vi "Inst_K2002.vi"(8 "error in":errorcluster, 10 "All Message Queues in":T1, 11 "AjustesPrevios in":refnum<class "AjustesPrevios.lvclass">) -> (0 "error out":errorcluster)   [LabVIEW 2019, in "AjustesPrevios.lvclass"]
uses:
  AjustesPrevios.lvclass
  QMH/Message Queue/All Message Queues.ctl
  QMH/Message Queue/Message Cluster.ctl
  AjustesPrevios.lvclass/AjustesPrevios.ctl
  <vilib>/Utility/error.llb/Error Cluster From Error Code.vi
  QMH/Message Queue/Enqueue Message (Single).vi
  <vilib>/ErrorRing/Error Ring.xnode
  QMH/Message Queue/Message Queue.lvlib
  Instrumento/Keithley2002/Keithley2002.lvclass
panel:
  out "All States":string[](array[string])
  out "Actual State":string
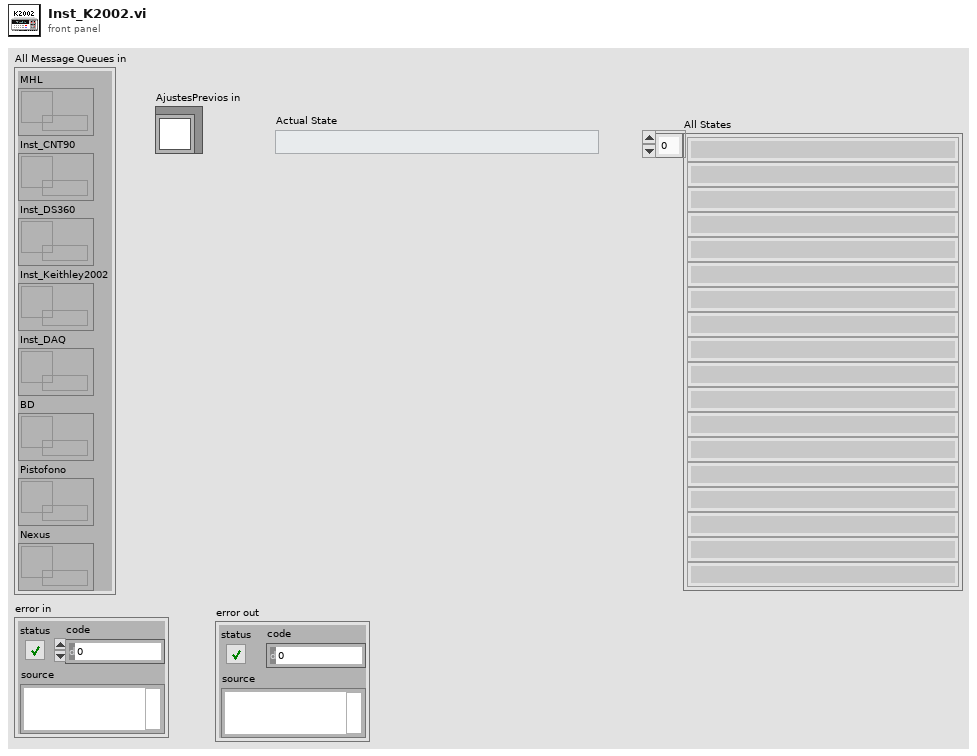
[diagram p1: front panel]
types:
  T1 = typedef "Message Queue.lvlib/All Message Queues.ctl" = cluster{"MHL":refnum<queue>, "Inst_CNT90":refnum<queue>, "Inst_DS360":refnum<queue>, "Inst_Keithley2002":refnum<queue>, "Inst_DAQ":refnum<queue>, "BD":refnum<queue>, "Pistofono":refnum<queue>, "Nexus":refnum<queue>}
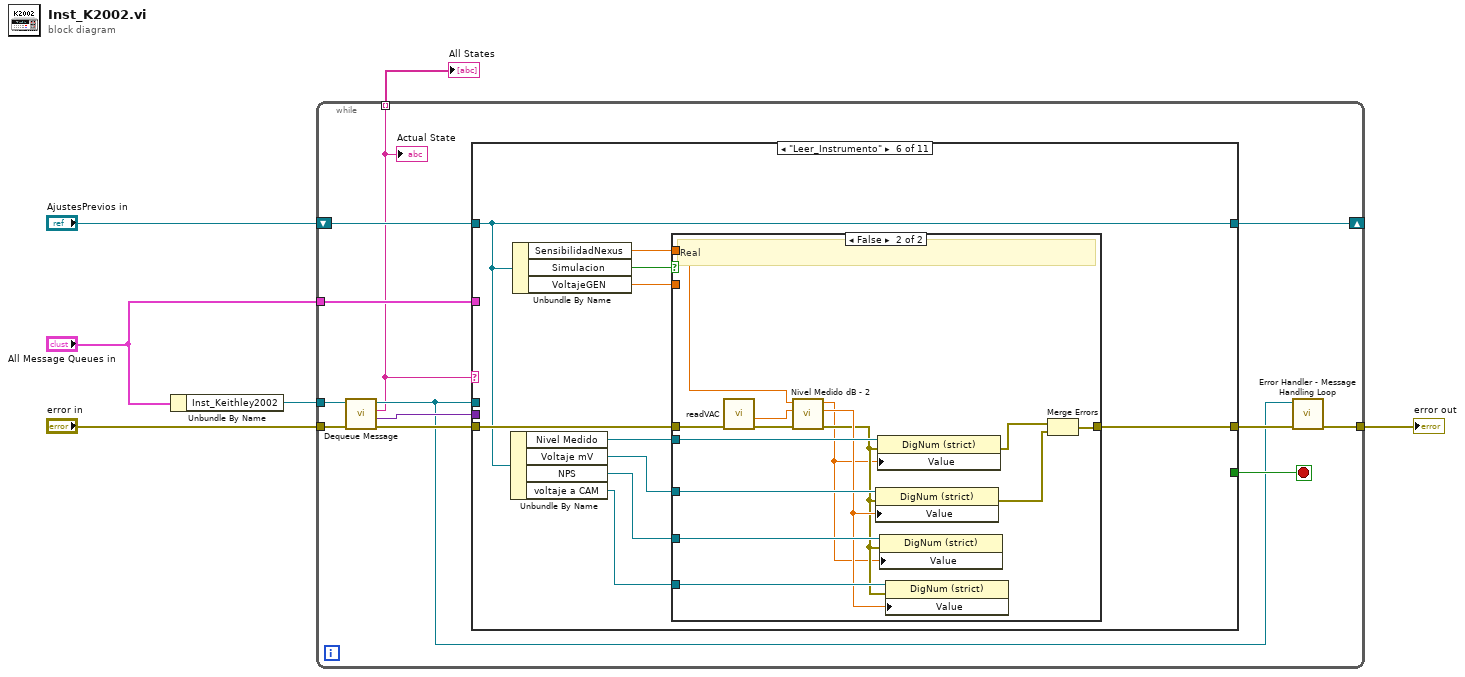
[diagram p0: block diagram]
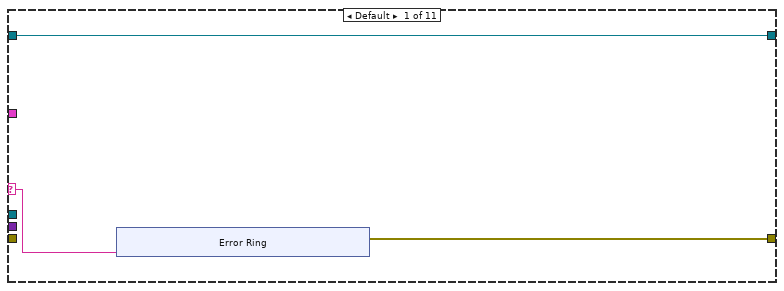
[diagram p2: hidden frame]
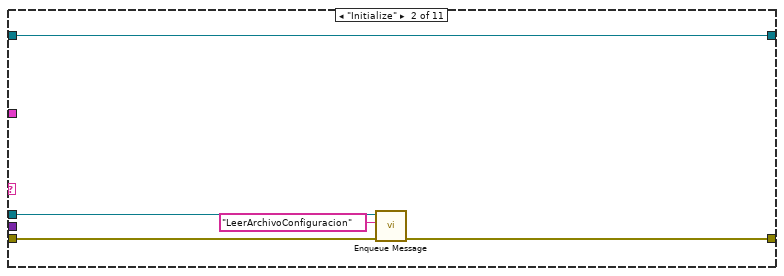
[diagram p3: hidden frame]
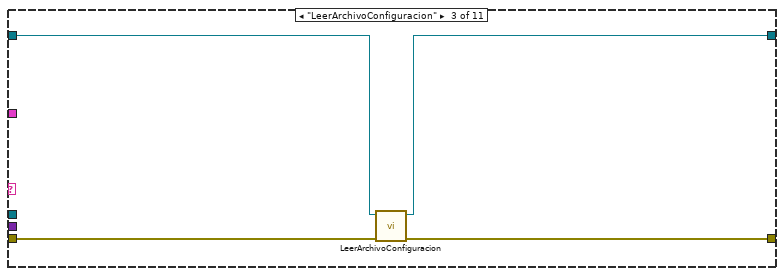
[diagram p4: hidden frame]
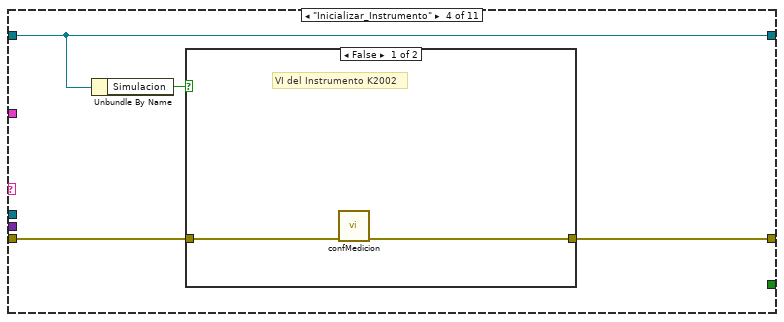
[diagram p5: hidden frame]
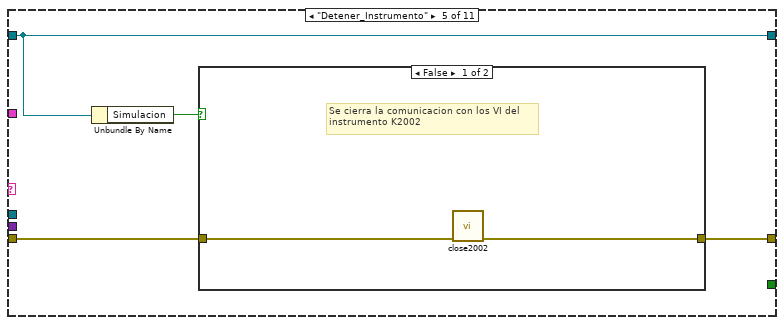
[diagram p7: hidden frame]
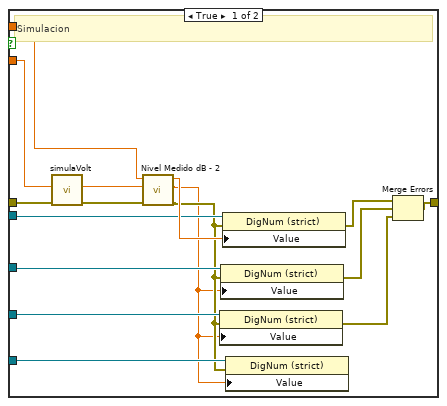
[diagram p9: hidden frame]
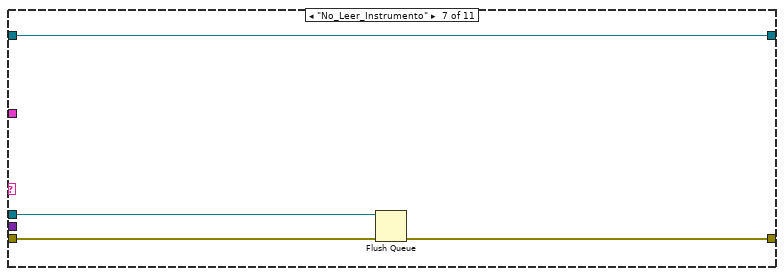
[diagram p10: hidden frame]
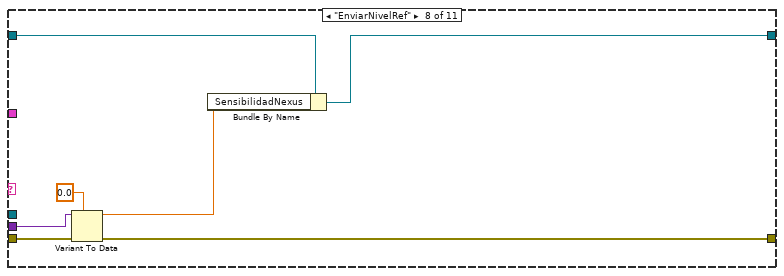
[diagram p11: hidden frame]
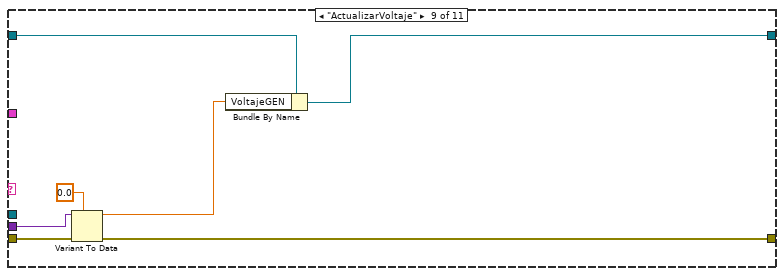
[diagram p12: hidden frame]
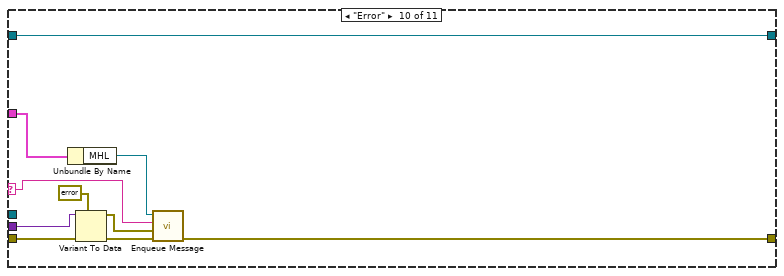
[diagram p13: hidden frame]
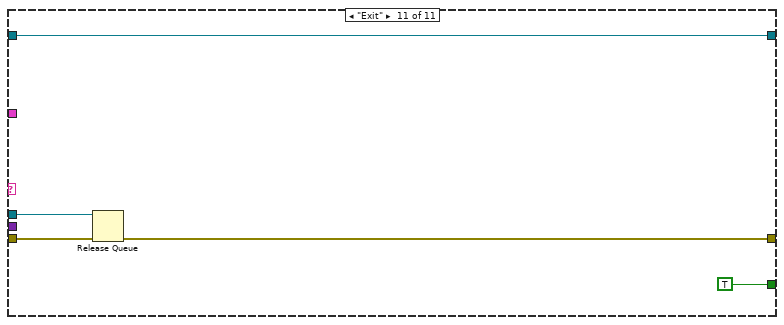
[diagram p14: hidden frame]
diagram:
  n1 = Unbundle By Name("All Message Queues in") -> ("Inst_Keithley2002"=w4:refnum<queue>)
  n2 = while {
    tunnel: "error in" -> [w18]
    tunnel: w4 -> [w17]
    tunnel: "All Message Queues in" -> [w16]
    tunnel: [w9] -> w2
    shift-right: [w12] -> _
    shift-left: "AjustesPrevios in" -> [w15]
    tunnel: [w7] -> w1 mode=indexing
    stop <- w11 stop-if-true
    n3 = call "Dequeue Message.vi"("error in (no error)"=w18, "Message Queue"=w17) -> ("error out"=w13:errorcluster, "Message Data"=w14:variant, "Message"=w7:string, "dup Message Queue"=w8:refnum<queue>)  [unwired: 6 in]
    "Actual State" <- w7
    n4 = case shown="\"Leer_Instrumento\"" w7 {
      selector: w7 -> [w21 _ _ _ _ _ _ _ _ w112 _]
      tunnel: w16 -> [_ _ _ _ _ _ _ _ _ w111 _]
      tunnel: w15 -> [w19 w33 w35 w38 w47 w57 w94 w97 w104 w119 w121]
      tunnel: w8 -> [_ w30 _ _ _ _ w92 _ _ _ w123]
      tunnel: w14 -> [_ _ _ _ _ _ _ w99 w106 w116 _]
      tunnel: w13 -> [_ w32 w37 w39 w45 w60 w95 w101 w108 w117 w124]
      tunnel: [w20 w31 w36 w41 w48 w59 w93 w102 w109 w114 w120] -> w10
      tunnel: [w19 w33 w34 w38 w47 w57 w94 w98 w105 w119 w121] -> w12
      tunnel: [_ _ _ _ _ _ _ _ _ _ TRUE] -> w11
      frame Default {
        n5 = xnode "Error Ring"("parameter 0"=w21) -> ("error out"=w20:errorcluster)
      }
      frame "Initialize" {
        n6 = call-poly "Enqueue Message.vi"("error in (no error)"=w32, "Message"="LeerArchivoConfiguracion", "Message Queue"=w30) -> ("error out"=w31:errorcluster)  [unwired: 7 in, 1 out]
      }
      frame "LeerArchivoConfiguracion" {
        n7 = call "LeerArchivoConfiguracion.vi"("error in"=w37, "AjustesPrevios in"=w35) -> ("error out"=w36:errorcluster, "AjustesPrevios out"=w34:refnum<class "AjustesPrevios.lvclass">)  [unwired: 8 in]
      }
      frame "Inicializar_Instrumento" {
        n8 = Unbundle By Name(w38) -> ("Simulacion"=w40:bool)
        n9 = case shown="False" w40 {
          tunnel: [w43 w44] -> w41
          tunnel: w39 -> [w42 w44]
          frame False {
            # "VI del Instrumento K2002"
            n10 = call "confMedicion.vi"("error in (no error)"=w42) -> ("error out"=w43:errorcluster)  [unwired: 9 in, 1 out]
          }
          frame True {
            # "Simulacion"
          }
        }
      }
      frame "Detener_Instrumento" {
        n11 = Unbundle By Name(w47) -> ("Simulacion"=w46:bool)
        n12 = case shown="False" w46 {
          tunnel: [w50 w51] -> w48
          tunnel: w45 -> [w49 w51]
          frame False {
            # "Se cierra la comunicacion con los VI del\ninstrumento K2002"
            n13 = call "close2002.vi"("error in (no error)"=w49) -> ("error out"=w50:errorcluster)  [unwired: 9 in, 1 out]
          }
          frame True {
            # "Simulacion"
          }
        }
      }
      frame "Leer_Instrumento" {
        n14 = Unbundle By Name(w57) -> ("Nivel Medido"=w56:refnum<vi>, "Voltaje mV"=w55:refnum<vi>, "NPS"=w53:refnum<vi>, "voltaje a CAM"=w52:refnum<vi>)
        n15 = Unbundle By Name(w57) -> ("SensibilidadNexus"=w58:dbl, "Simulacion"=w61:bool, "VoltajeGEN"=w54:dbl)
        n16 = case shown="False" w61 {
          tunnel: [w71 w85] -> w59
          tunnel: w60 -> [w77 w91]
          tunnel: w58 -> [w75 w88]
          tunnel: w56 -> [w69 w87]
          tunnel: w55 -> [w68 w86]
          tunnel: w54 -> [w67 _]
          tunnel: w53 -> [w66 w82]
          tunnel: w52 -> [w64 w81]
          frame True {
            # "Simulacion"
            n17 = call "simulaVolt.vi"("error in (no error)"=w77, "volt in"=w67) -> ("error out"=w76:errorcluster, "volt out"=w74:dbl)  [unwired: 7 in, 1 out]
            n18 = call "Nivel Medido dB - 2.vi"("error in (no error)"=w76, "voltaje_medido"=w74, "Sensibilidad"=w75) -> ("error out"=w63:errorcluster, "voltaje mV"=w62:dbl, "Nivel Medido [dB]"=w70:dbl)  [unwired: 6 in]
            n19 = property class="DigNum (strict)"(reference=w66, error in=w63, "Value"=w62) -> (error out=w65:errorcluster)  [unwired: 1 out]
            n20 = property class="DigNum (strict)"(reference=w68, error in=w63, "Value"=w62) -> (error out=w72:errorcluster)  [unwired: 1 out]
            n21 = property class="DigNum (strict)"(reference=w69, error in=w63, "Value"=w70) -> (error out=w73:errorcluster)  [unwired: 1 out]
            n22 = property class="DigNum (strict)"(reference=w64, error in=w63, "Value"=w62) -> ()  [unwired: 2 out]
            n23 = Merge Errors(w73, w72, w65) -> (w71:errorcluster)
          }
          frame False {
            # "Real"
            n24 = call "readVAC.vi"("error in (no error)"=w91) -> ("error out"=w90:errorcluster, "medicion"=w89:dbl)  [unwired: 7 in, 2 out]
            n25 = call "Nivel Medido dB - 2.vi"("error in (no error)"=w90, "voltaje_medido"=w89, "Sensibilidad"=w88) -> ("error out"=w79:errorcluster, "voltaje mV"=w80:dbl, "Nivel Medido [dB]"=w78:dbl)  [unwired: 6 in]
            n26 = property class="DigNum (strict)"(reference=w86, error in=w79, "Value"=w80) -> (error out=w83:errorcluster)  [unwired: 1 out]
            n27 = property class="DigNum (strict)"(reference=w87, error in=w79, "Value"=w78) -> (error out=w84:errorcluster)  [unwired: 1 out]
            n28 = property class="DigNum (strict)"(reference=w82, error in=w79, "Value"=w78) -> ()  [unwired: 2 out]
            n29 = property class="DigNum (strict)"(reference=w81, error in=w79, "Value"=w80) -> ()  [unwired: 2 out]
            n30 = Merge Errors(w84, w83) -> (w85:errorcluster)
          }
        }
      }
      frame "No_Leer_Instrumento" {
        n31 = Flush Queue(queue=w92, error in (no error)=w95) -> (error out=w93:errorcluster)  [unwired: 2 out]
      }
      frame "EnviarNivelRef" {
        n32 = Variant To Data(error in=w101, type=0.0, Variant=w99) -> (data=w96:dbl, error out=w102:errorcluster)
        n33 = Bundle By Name(cluster=w97, "SensibilidadNexus"=w96) -> (w98:refnum<class "AjustesPrevios.lvclass">)
      }
      frame "ActualizarVoltaje" {
        n34 = Variant To Data(error in=w108, type=0.0, Variant=w106) -> (data=w103:dbl, error out=w109:errorcluster)
        n35 = Bundle By Name(cluster=w104, "VoltajeGEN"=w103) -> (w105:refnum<class "AjustesPrevios.lvclass">)
      }
      frame "Error" {
        n36 = Unbundle By Name(w111) -> ("MHL"=w110:refnum<queue>)
        n37 = Variant To Data(error in=w117, type=errorcluster {"status"=FALSE, "code"=0, "source"=""} ("error constant"), Variant=w116) -> (data=w113:errorcluster, error out=w115:errorcluster)
        n38 = call-poly "Enqueue Message.vi"("error in (no error)"=w115, "Message Data"=w113, "Message"=w112, "Message Queue"=w110) -> ("error out"=w114:errorcluster)  [unwired: 6 in, 1 out]
      }
      frame "Exit" {
        n39 = Release Queue(queue=w123, error in (no error)=w124) -> (error out=w120:errorcluster)  [unwired: 1 in, 2 out]
      }
    }
    n40 = call "Error Handler - Message Handling Loop.vi"("error in (no error)"=w10, "Message Queue"=w8) -> ("dup error in"=w9:errorcluster)  [unwired: 8 in, 1 out]
  }
  "error out" <- w2
  "All States" <- w1
